vi "Test_wykrywania_konfiguracji.vi"(8 "error in (no error)":errorcluster, 11 "Konfiguracja in":path=path "C:/Users/user/Documents/Rudpol2/Konfiguracja") -> (0 "error out":errorcluster, 2 "Plik":string)   [LabVIEW 2014]
doc: "Wybiera plik konfiguracyjny dla kanałów analogowych\ndla podłączonego rejestratora"
uses:
  <vilib>/Utility/miscctls.llb/LVStringsAndValuesArrayTypeDef_U16.ctl
panel:
  in  "Urzadzenie":u16(ring) caption="Wybierz Urządzenie" items=["REJESTRATOR 1", "REJESTRATOR 10", "REJESTRATOR 2", "REJESTRATOR 3"]
  in  "OK Button":bool
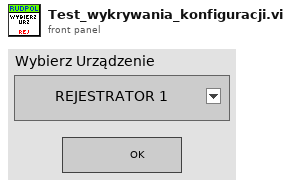
[diagram p1: front panel]
types:
  T1 = typedef "LVStringsAndValuesArrayTypeDef_U16.ctl" = cluster{"String":string, "Value":u16}[]
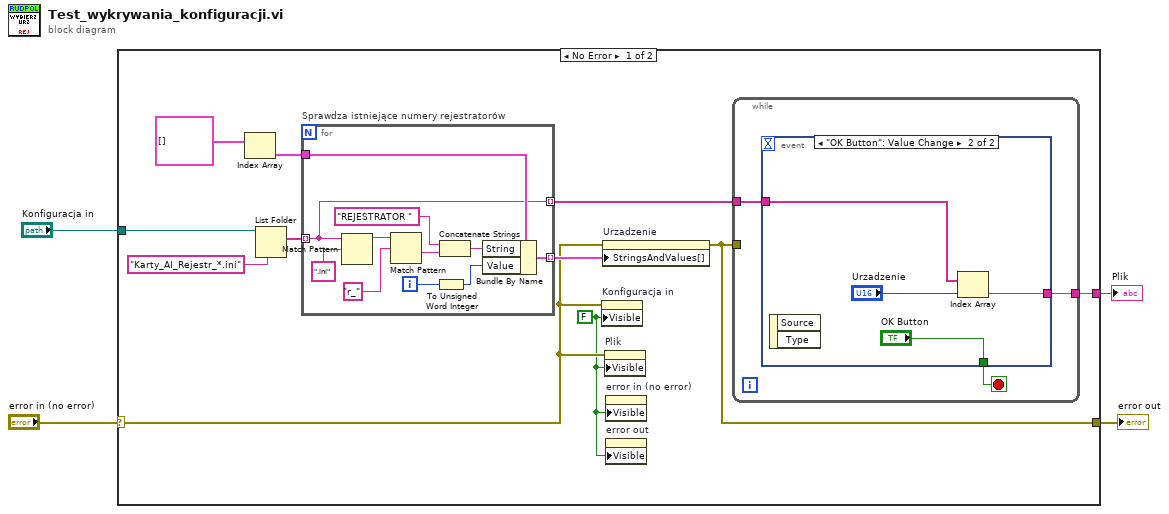
[diagram p0: block diagram]
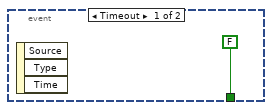
[diagram p2: hidden frame]
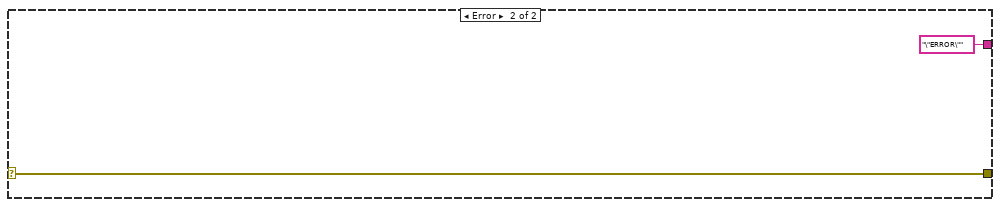
[diagram p3: hidden frame]
diagram:
  n1 = case shown="No Error" "error in (no error)" {
    selector: "error in (no error)" -> [w7 w35]
    tunnel: "Konfiguracja in" -> [w14 _]
    tunnel: [w9 "\"ERROR\""] -> w3
    tunnel: [w6 w35] -> w1
    frame No Error {
      w5 = FALSE ("Visible")
      n2 = Index Array(array=T1 [] ("Strings And Values []")) -> (element=w12:cluster{"String":string, "Value":u16})  [unwired: 1 in]
      n3 = List Folder(path=w14, pattern="Karty_AI_Rejestr_*.ini") -> (filenames=w8:string[])  [unwired: 2 in, 3 out]
      n4 = for "Sprawdza istniejące numery rejestratorów" {
        tunnel: w8 -> [w24] mode=indexing
        tunnel: [w29] -> w10 mode=indexing
        tunnel: w12 -> [w25]
        tunnel: [w24] -> w11 mode=indexing
        i -> [w28]
        n5 = Match Pattern(string=w24, regular expression=".ini") -> (before substring=w33:string)  [unwired: 1 in, 3 out]
        n6 = Match Pattern(string=w33, regular expression="r_") -> (after substring=w31:string)  [unwired: 1 in, 3 out]
        n7 = To Unsigned Word Integer(number=w28) -> (unsigned 16bit integer=w27:u16)
        n8 = Concatenate Strings("REJESTRATOR " ("regular expression"), w31) -> (w26:string)
        n9 = Bundle By Name(cluster=w25, "String"=w26, "Value"=w27) -> (w29:cluster{"String":string, "Value":u16})
      }
      n10 = property on="Konfiguracja in" class="Path"(error in=w7, "Visible"=w5) -> ()  [unwired: 1 in, 2 out]
      n11 = property on="Urzadzenie" class="Ring (strict)"(error in=w7, "StringsAndValues[]"=w10) -> (error out=w6:errorcluster)  [unwired: 1 in, 1 out]
      n12 = property on="Plik" class="Str"(error in=w7, "Visible"=w5) -> ()  [unwired: 1 in, 2 out]
      n13 = property on="error in (no error)" class="Clust (strict)"("Visible"=w5) -> ()  [unwired: 2 in, 2 out]
      n14 = property on="error out" class="Clust (strict)"("Visible"=w5) -> ()  [unwired: 2 in, 2 out]
      n15 = while {
        tunnel: w11 -> [w17]
        tunnel: w6 -> [_]
        tunnel: [w16] -> w9
        stop <- w18 stop-if-true
        n16 = event shown="[1] \"OK Button\": Value Change" {
          selector: _ -> [_ _]
          dyn-events: _ -> [_ _]
          timeout: _ -> [_ _]
          tunnel: [FALSE ("OK Button") "OK Button"] -> w18
          tunnel: w17 -> [_ w21]
          tunnel: [_ w20] -> w16
          event Timeout {
            n17 = event-data() -> ()  [unwired: 1 in, 3 out]
          }
          event "OK Button": Value Change {
            n18 = event-data() -> ()  [unwired: 1 in, 2 out]
            n19 = Index Array(array=w21, index="Urzadzenie") -> (element=w20:string)
          }
        }
      }
    }
    frame Error {
    }
  }
  "Plik" <- w3
  "error out" <- w1
